vi "PowerSupplyBuildTags.vi"(8 "error in (no error)":errorcluster, 10 "Config":T2, 11 "ModuleID":string) -> (0 "error out":errorcluster, 3 "Tag Refs":T1)   [LabVIEW 2020, in "PowerSupply.lvlib"]
uses:
  PowerSupply.lvlib
  <vilib>/Tag Engine/Tag/Tag.lvclass
  <vilib>/Tag Engine/Tag/Tag.lvclass/Tag.ctl
  ac7728c8-b444-4933-8733-8bfc8ca51d41.vi
  7ccb3626-d3b5-4d34-938e-bee8e8a4e942.vi
  45a23698-ef1e-48a7-a600-587e830a9218.vi
  b3d22764-8541-49ad-a00f-f3f19130bb0e.vi
  <vilib>/Tag Engine/Tag/Write Max.vi
  <vilib>/Tag Engine/Tag/Write Min.vi
  <vilib>/Tag Engine/Tag/Construct.vi
  <vilib>/Tag Engine/Core/Get Delimiter.vi
  <vilib>/Utility/error.llb/Error Cluster From Error Code.vi
  <vilib>/Tag Engine/Tag/Set Properties from Initial.vi
  <vilib>/Tag Engine/Core/Add Tag.vi
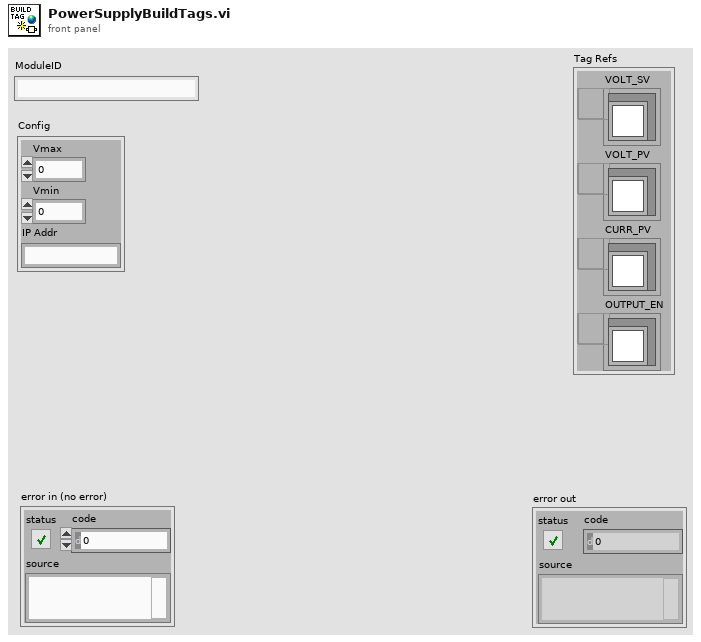
[diagram p1: front panel]
types:
  T1 = cluster{"VOLT_SV":refnum<data-value>, "VOLT_PV":refnum<data-value>, "CURR_PV":refnum<data-value>, "OUTPUT_EN":refnum<data-value>}
  T2 = cluster{"Vmax":dbl, "Vmin":dbl, "IP Addr":string}
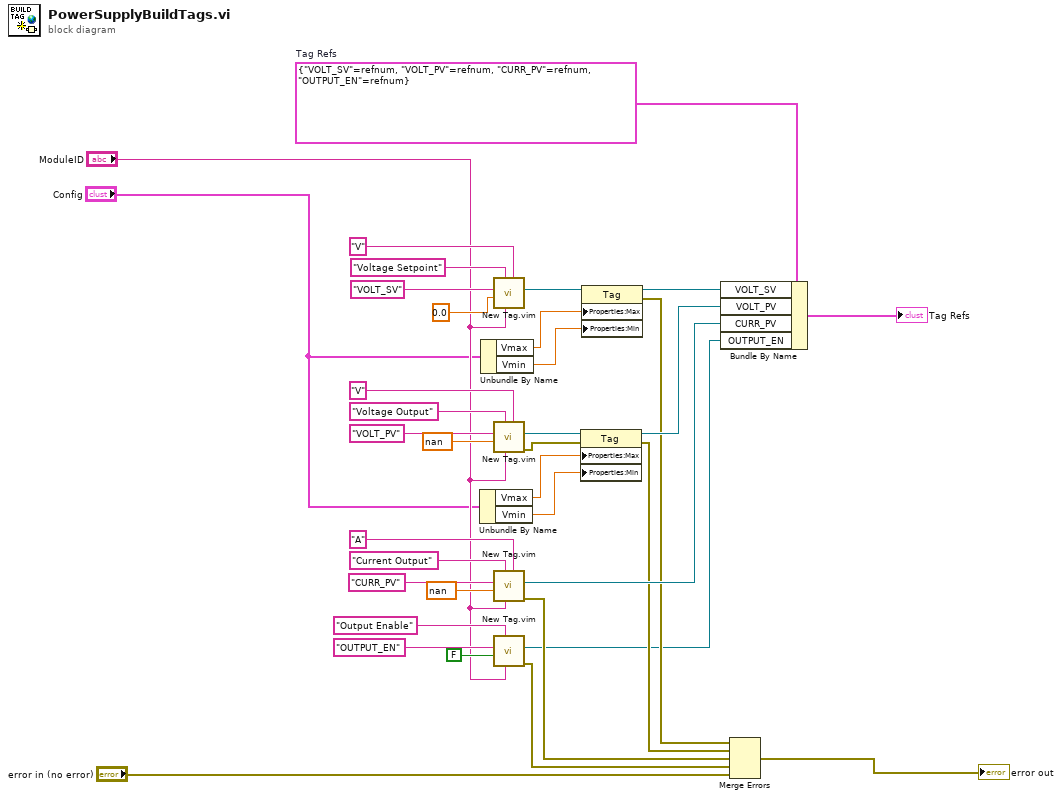
[diagram p0: block diagram]
diagram:
  w5 = T1 {"VOLT_SV"=refnum, "VOLT_PV"=refnum, "CURR_PV"=refnum, "OUTPUT_EN"=refnum}  # Tag Refs
  n1 = Unbundle By Name("Config") -> ("Vmax"=w24:dbl, "Vmin"=w23:dbl)
  n2 = Unbundle By Name("Config") -> ("Vmax"=w34:dbl, "Vmin"=w33:dbl)
  n3 = call "New Tag.vim"("Units (none)"="V", "Namespace"="ModuleID", "Description (none)"="Voltage Setpoint", "Initial Value"=0.0, "Tag Name"="VOLT_SV") -> ("Tag Ref out"=w35:refnum<data-value>)  [unwired: 5 in, 1 out]
  n4 = call "New Tag.vim"("Units (none)"="V", "Namespace"="ModuleID", "Description (none)"="Voltage Output", "Initial Value"=nan, "Tag Name"="VOLT_PV") -> ("error out"=w9:errorcluster, "Tag Ref out"=w25:refnum<data-value>)  [unwired: 5 in]
  n5 = call "New Tag.vim"("Units (none)"="A", "Namespace"="ModuleID", "Description (none)"="Current Output", "Initial Value"=nan, "Tag Name"="CURR_PV") -> ("error out"=w10:errorcluster, "Tag Ref out"=w16:refnum<data-value>)  [unwired: 5 in]
  n6 = call "New Tag.vim"("Namespace"="ModuleID", "Description (none)"="Output Enable", "Initial Value"=FALSE, "Tag Name"="OUTPUT_EN") -> ("error out"=w11:errorcluster, "Tag Ref out"=w6:refnum<data-value>)  [unwired: 6 in]
  n7 = property class="Tag"(reference=w25, error in=w9, "Properties:Max"=w24, "Properties:Min"=w23) -> (reference out=w17:refnum<data-value>, error out=w8:errorcluster)
  n8 = property class="Tag"(reference=w35, "Properties:Max"=w34, "Properties:Min"=w33) -> (reference out=w18:refnum<data-value>, error out=w7:errorcluster)  [unwired: 1 in]
  n9 = Bundle By Name(cluster=w5, "VOLT_SV"=w18, "VOLT_PV"=w17, "CURR_PV"=w16, "OUTPUT_EN"=w6) -> (→"Tag Refs":T1)
  n10 = Merge Errors(w7, w8, w10, w11, "error in (no error)") -> (→"error out":errorcluster)
